vi "HV VSet Multi.vi"(8 "Voltage":string[](array[string]), 11 "Channel":string[](array[string])) -> (0 "Output":string[](array[string]))   [LabVIEW 2018, in "HV QMH.lvlib"]
uses:
  HV QMH.lvlib
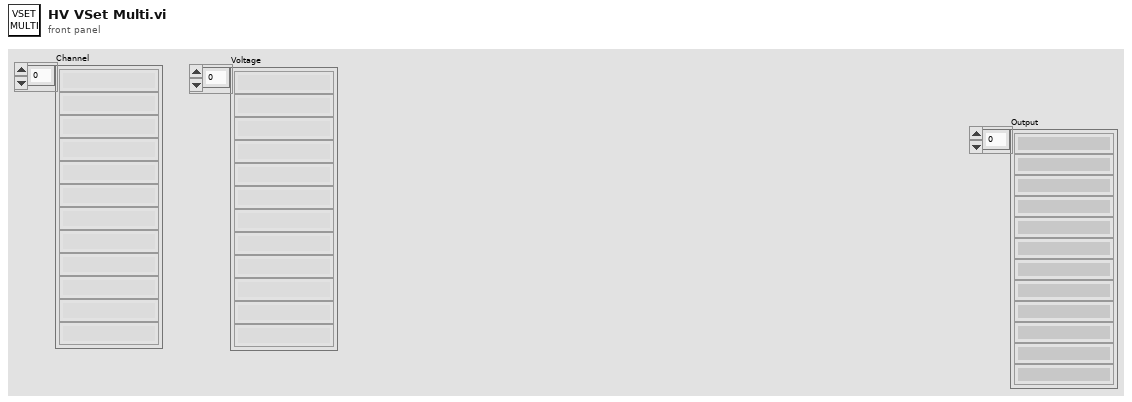
[diagram p1: front panel]
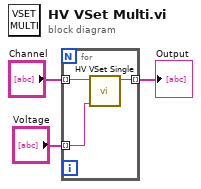
[diagram p0: block diagram]
diagram:
  n1 = for {
    tunnel: "Channel" -> [w6] mode=indexing
    tunnel: "Voltage" -> [w5] mode=indexing
    tunnel: [w4] -> w1 mode=indexing
    n2 = call "HV VSet Single.vi"("Voltage"=w5, "Channel"=w6) -> ("standard output"=w4:string)  [unwired: 9 in]
  }
  "Output" <- w1
